vi "Calculate Add Tab Button Position.vi"(8 "error in":errorcluster, 10 "Tab Control Reference In":refnum<vi>, 11 "Add Tab Button Reference In":refnum<vi>) -> (0 "error out":errorcluster, 1 "Button Position":i32, 2 "Add Tab Button Reference Out":refnum<vi>, 3 "Tab Control Reference Out":refnum<vi>)   [LabVIEW 2017, in "DTacq Plot Display Library.lvlib"]
uses:
  DTacq Plot Display Library.lvlib
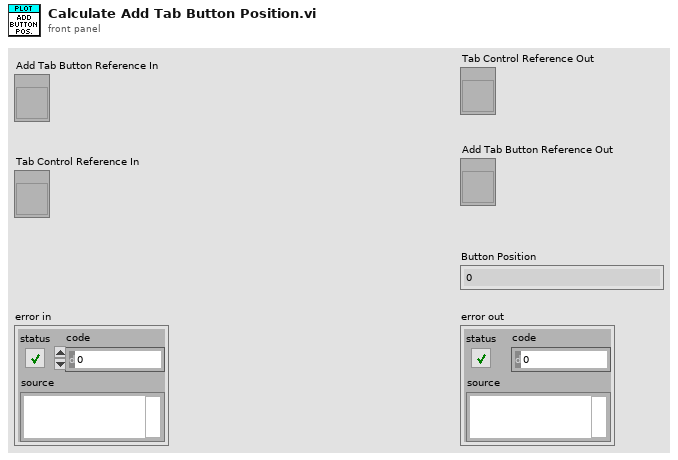
[diagram p1: front panel]
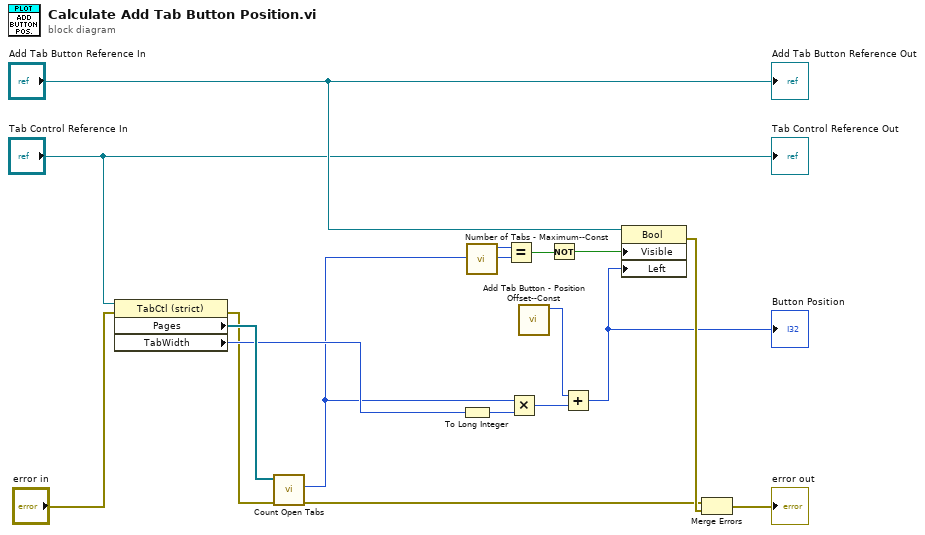
[diagram p0: block diagram]
diagram:
  n1 = property class="TabCtl (strict)"(reference="Tab Control Reference In", error in="error in") -> (error out=w2:errorcluster, "Pages"=w9:refnum<vi>[], "TabWidth"=w8:u32)  [unwired: 1 out]
  n2 = call "Count Open Tabs.vi"("error in"=w2, "Tab Pages References In"=w9) -> ("error out"=w3:errorcluster, "Number of Open Tabs"=w1:i32)  [unwired: 7 in, 1 out]
  n3 = To Long Integer(number=w8) -> (32bit integer=w12:i32)
  n4 = call "Number of Tabs - Maximum--Const.vi"() -> ("Maximum Tabs"=w6:i32)  [unwired: 11 in]
  n5 = Equal?(x=w6, y=w1) -> (x = y?=w5:bool)
  n6 = Multiply(x=w1, y=w12) -> (x*y=w17:i32)
  n7 = call "Add Tab Button - Position Offset--Const.vi"() -> ("Position Offset"=w10:i32)  [unwired: 11 in]
  n8 = Not(x=w5) -> (.not. x?=w4:bool)
  n9 = Add(x=w10, y=w17) -> (x+y=w7:i32)
  "Button Position" <- w7
  n10 = property class="Bool"(reference="Add Tab Button Reference In", "Visible"=w4, "Left"=w7) -> (error out=w14:errorcluster)  [unwired: 1 in, 1 out]
  n11 = Merge Errors(w3, w14) -> (→"error out":errorcluster)
  "Tab Control Reference Out" <- "Tab Control Reference In"
  "Add Tab Button Reference Out" <- "Add Tab Button Reference In"
